vi "KeyWords.vi"() -> (2 "%[hex] Code":string[](array[string])=["%2D%3E%7C", "%2D%3E", "%2D%40", "%2D%26", "%3C%2D", "%0D", "%0A", "%09", "%5C", "%23"], 3 "Source":string[](array[string])=["->|", "->", "-@", "-&", "<-", "\r", "\n", "\t", "\\", "#"])   [LabVIEW 2014, in "JKI State Machine++.lvlib"]
uses:
  JKI State Machine++.lvlib
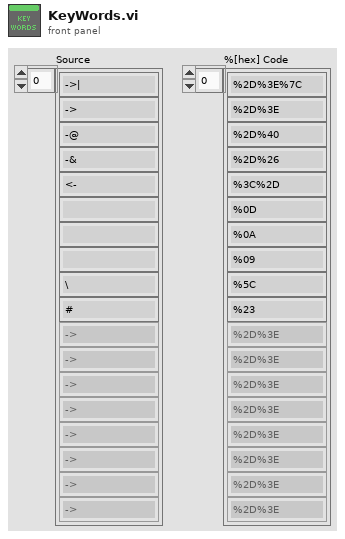
[diagram p1: front panel]
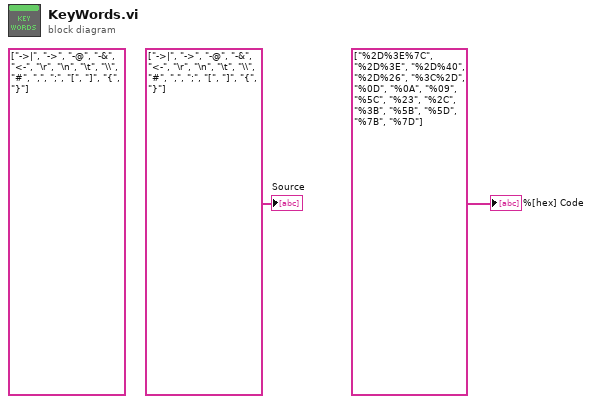
[diagram p0: block diagram]
diagram:
  (unwired) string[] ["->|", "->", "-@", "-&", "<-", "\r", "\n", "\t", "\\", "#", ",", ";", "[", "]", "{", "}"]
  "%[hex] Code" <- string[] ["%2D%3E%7C", "%2D%3E", "%2D%40", "%2D%26", "%3C%2D", "%0D", "%0A", "%09", "%5C", "%23", "%2C", "%3B", "%5B", "%5D", "%7B", "%7D"]
  "Source" <- string[] ["->|", "->", "-@", "-&", "<-", "\r", "\n", "\t", "\\", "#", ",", ";", "[", "]", "{", "}"]
